vi "Stats.vi"(4 "Scan Period":dbl, 6 "Present scan array":dbl[](array[numeric]), 8 "Ch Description":T1 {"Duty" format="%.0b"; "D" format="%#_5g"; "C" format="%#_5g"; "B" format="%#_5g"; "A" format="%#_5g"}, 9 "Ch names":string[](array[string])) -> (0 "String":string, 1 "Stat":dbl, 3 "HelpText":string="\"A\" Warn if above this value\n\"B\" Warn if below this value\n\"C\" Hysteresis margin\n\"D\" is the averaging time in minutes\n\nWrite Channel name to check in the box above \"Comparator\"")   [LabVIEW 2015]
uses:
  ADAM Client/Sub VIs/ADAM Controls/Ch_description_ADAM.ctl
  ADAM Client/Sub VIs/ADAM Controls/Module_type_ADAM.ctl
  ADAM Client/Sub VIs/ADAM Controls/Function_ADAM.ctl
  ADAM Client/Sub VIs/ADAM Controls/Channel_State.ctl
  ADAM Client/Sub VIs/ADAM Controls/Calib_type_ADAM.ctl
  ADAM Client/Sub VIs/ADAM Controls/Address.ctl
  ADAM_Global.vi
  <vilib>/Analysis/NI_AALBase.lvlib
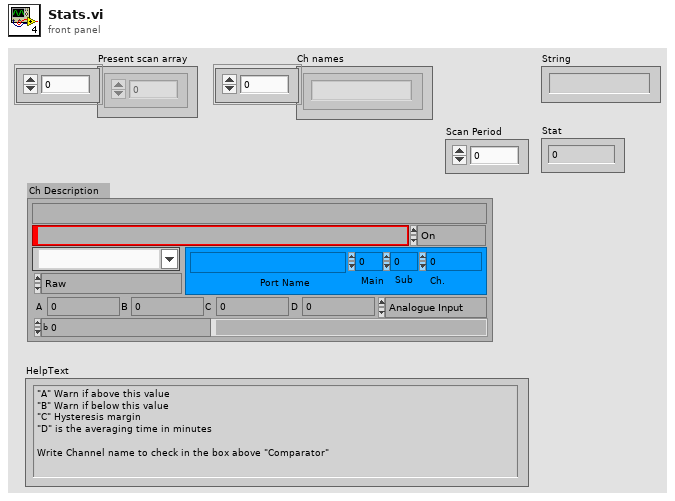
[diagram p1: front panel]
types:
  T1 = typedef "Ch_description_ADAM.ctl" = cluster{"Ch Name":string, "Type":T2, "Function":T3, "Ch State":T4, "Calibration type":T5, "A":dbl, "B":dbl, "C":dbl, "D":dbl, "Comments":string, "Address":T6, "String":string, "Duty":u16}
  T2 = typedef "Module_type_ADAM.ctl" = string
  T3 = typedef "Function_ADAM.ctl" = enum16{"Analogue Input", "Digital Input", "Event counter", "Event rate", "Analogue Output", "Digital Output", "Relay Output"}
  T4 = typedef "Channel_State.ctl" = enum16{"On", "Off", "Always On", "Always Off"}
  T5 = typedef "Calib_type_ADAM.ctl" = enum16{"Raw", "Bx + A", "Cx^2 + Bx + A", "Dx^3 + Cx^2 + Bx + A", "In Band", "Hi-Tec Q", "Hi-Tec M_dot", "Text"}
  T6 = typedef "Address.ctl" = cluster{"Main":i32, "Ch.":i32, "Sub":i32, "Port Name":string}
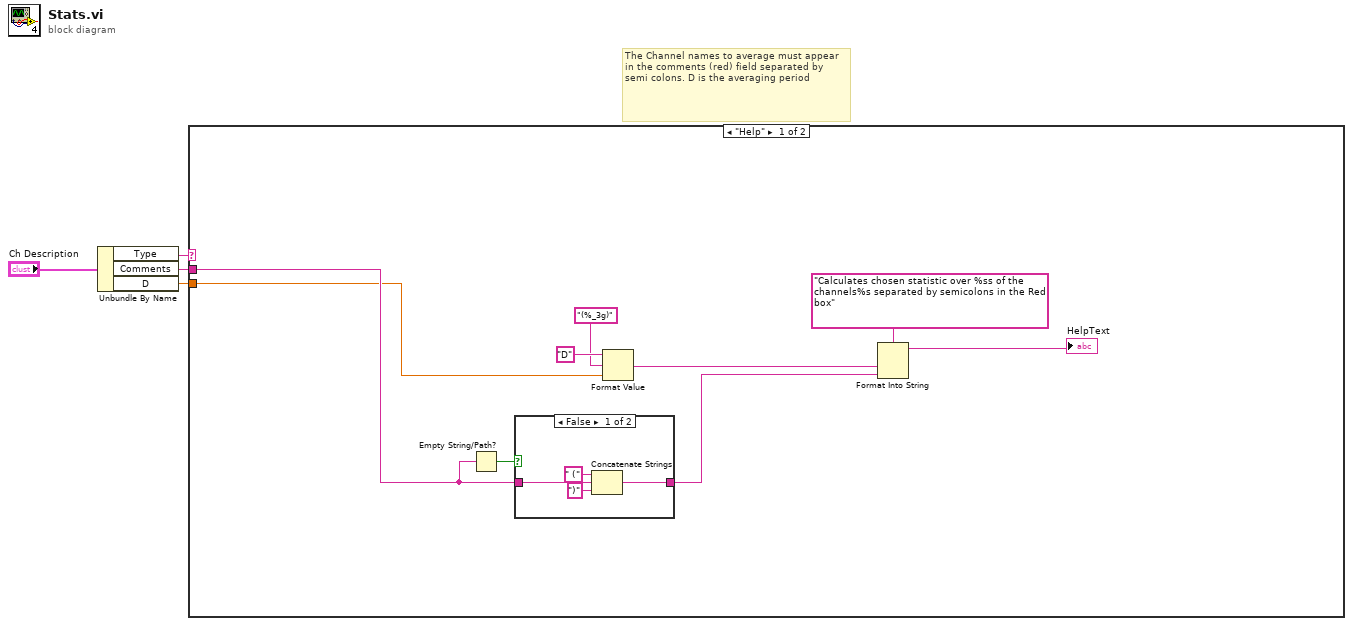
[diagram p0: block diagram]
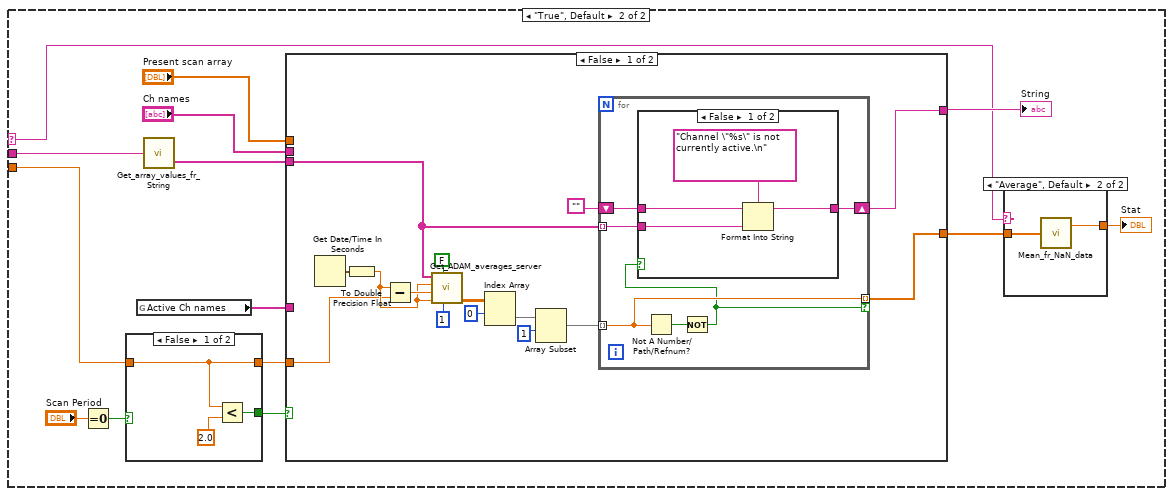
[diagram p3: hidden frame]
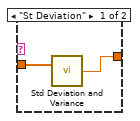
[diagram p4: hidden frame]
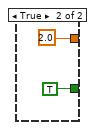
[diagram p5: hidden frame]
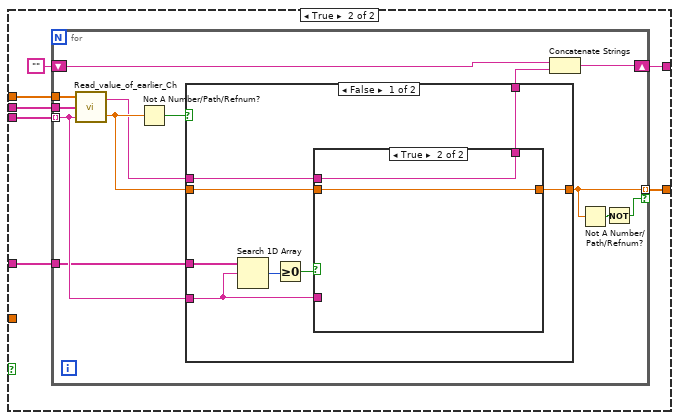
[diagram p7: hidden frame]
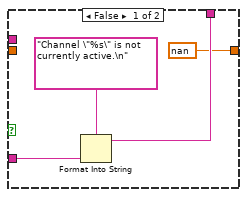
[diagram p8: hidden frame]
diagram:
  # "The Channel names to average must appear in the comments (red) field separated by semi colons. D is the averaging period"
  n1 = Unbundle By Name("Ch Description") -> ("Type"=w2:T2, "Comments"=w4:string, "D"=w1:dbl)
  n2 = case shown="\"Help\"" w2 {
    selector: w2 -> [_ w19]
    tunnel: w4 -> [w11 w21]
    tunnel: w1 -> [w6 w20]
    frame "Help" {
      n3 = Empty String/Path?(string/path=w11) -> (empty?=w13:bool)
      n4 = case shown="False" w13 {
        tunnel: [w16 w18] -> w9
        tunnel: w11 -> [w17 w18]
        frame False {
          n5 = Concatenate Strings(" (" ("string"), w17, ")" ("string")) -> (w16:string)
        }
        frame True {
        }
      }
      n6 = Format Value(string ("")="D", format string="(%_3g)", value (0)=w6) -> (output string=w5:string)
      n7 = Format Into String(format string="Calculates chosen statistic over %ss of the channels%s separated by semicolons in the Red box", w5, w9) -> (resulting string=→"HelpText":string)  [unwired: 2 in, 1 out]
    }
    frame "True", Default {
      n8 = Equal To 0?(x="Scan Period") -> (x = 0?=w29:bool)
      n9 = case shown="False" w29 {
        tunnel: [w38 TRUE] -> w26
        tunnel: [w37 2.0 ("A")] -> w27
        tunnel: w20 -> [w37 _]
        frame False {
          n10 = Less?(x=w37, y=2.0) -> (x < y?=w38:bool)
        }
        frame True {
        }
      }
      n11 = global read "ADAM_Global.vi" "Active Ch names"() -> (w25:string[])
      n12 = call "Get_array_values_fr_String.vi"("String Value"=w21) -> ("String array"=w24:string[])  [unwired: 1 out]
      n13 = case shown="False" w26 {
        tunnel: "Ch names" -> [_ w74]
        tunnel: "Present scan array" -> [_ w73]
        tunnel: w24 -> [w44 w72]
        tunnel: [w42 w70] -> w30
        tunnel: w25 -> [_ w69]
        tunnel: [w45 w68] -> w31
        tunnel: w27 -> [w46 _]
        frame False {
          n14 = Get Date/Time In Seconds() -> (seconds since 1Jan1904=w56:timestamp)
          n15 = To Double Precision Float(number=w56) -> (double precision float=w54:dbl)
          n16 = Subtract(x=w54, y=w46) -> (x-y=w55:dbl)
          n17 = call "Get_ADAM_averages_server.vi"("No of averages"=1, "All Active Channels"=FALSE, "End time"=w54, "Start time"=w55, "Clients time"=w54, "ADAM Ch Names"=w44) -> ("DBL values"=w51:dbl[][])  [unwired: 4 out]
          n18 = Index Array(array=w51, index (row)=0) -> (element=w48:dbl[])  [unwired: 1 in]
          n19 = Array Subset(array=w48, index=1) -> (w47:dbl[])  [unwired: 1 in]
          n20 = for {
            tunnel: w47 -> [w62] mode=indexing
            tunnel: [w62] -> w45 mode=indexing if=w60
            tunnel: w44 -> [w59] mode=indexing
            shift-right: [w57] -> w42
            shift-left: "" -> [w58]
            n21 = Not A Number/Path/Refnum?(number/path/refnum=w62) -> (NaN/Path/Refnum?=w61:bool)
            n22 = Not(x=w61) -> (.not. x?=w60:bool)
            n23 = case shown="False" w60 {
              tunnel: w59 -> [w65 _]
              tunnel: w58 -> [w64 w67]
              tunnel: [w63 w67] -> w57
              frame False {
                n24 = Format Into String(format string="Channel \"%s\" is not currently active.\n", initial string=w64, w65) -> (resulting string=w63:string)  [unwired: 1 in, 1 out]
              }
              frame True {
              }
            }
          }
        }
        frame True {
          n25 = for {
            tunnel: w74 -> [w87]
            tunnel: w73 -> [w86]
            tunnel: w72 -> [w83] mode=indexing
            shift-right: [w84] -> w70
            shift-left: "" -> [w85]
            tunnel: [w77] -> w68 mode=indexing if=w75
            tunnel: w69 -> [w78]
            n26 = call "Read_value_of_earlier_Ch.vi"("Desired Ch to Read"=w83, "Ch names"=w87, "Present scan array"=w86) -> ("Value"=w81:dbl, "Scan comment"=w80:string)  [unwired: 1 in]
            n27 = Not A Number/Path/Refnum?(number/path/refnum=w81) -> (NaN/Path/Refnum?=w82:bool)
            n28 = case shown="False" w82 {
              tunnel: w83 -> [w90 _]
              tunnel: [w93 w103] -> w77
              tunnel: w81 -> [w92 w103]
              tunnel: [w95 w102] -> w79
              tunnel: w80 -> [w94 w102]
              tunnel: w78 -> [w91 _]
              frame False {
                n29 = Search 1D Array(1D array=w91, element=w90) -> (index of element=w88:i32)  [unwired: 1 in]
                n30 = Greater Or Equal To 0?(x=w88) -> (x >= 0?=w89:bool)
                n31 = case shown="True" w89 {
                  tunnel: w90 -> [w99 _]
                  tunnel: [w98 w101] -> w95
                  tunnel: w94 -> [_ w101]
                  tunnel: [nan w100] -> w93
                  tunnel: w92 -> [_ w100]
                  frame False {
                    n32 = Format Into String(format string="Channel \"%s\" is not currently active.\n", w99) -> (resulting string=w98:string)  [unwired: 2 in, 1 out]
                  }
                  frame True {
                  }
                }
              }
              frame True {
              }
            }
            n33 = Concatenate Strings(w85, w79) -> (w84:string)
            n34 = Not A Number/Path/Refnum?(number/path/refnum=w77) -> (NaN/Path/Refnum?=w76:bool)
            n35 = Not(x=w76) -> (.not. x?=w75:bool)
          }
        }
      }
      "String" <- w30
      n36 = case shown="\"Average\", Default" w19 {
        tunnel: [w33 w36] -> w32
        tunnel: w31 -> [w34 w35]
        frame "St Deviation" {
          n37 = call <vilib>:"Std Deviation and Variance.vi"("X"=w34) -> ("standard deviation"=w33:dbl)  [unwired: 1 in, 2 out]
        }
        frame "Average", Default {
          n38 = call "Mean_fr_NaN_data.vi"("Data"=w35) -> ("Mean value"=w36:dbl)  [unwired: 1 out]
        }
      }
      "Stat" <- w32
    }
  }
